vi "Wait for Message.vi"(1 "gui notification":string, 2 "cases to ignore":string[](array[string]), 3 "last state":string, 4 "acquisition state name":string) -> (0 "wait for notification?":bool)   [LabVIEW 2020]
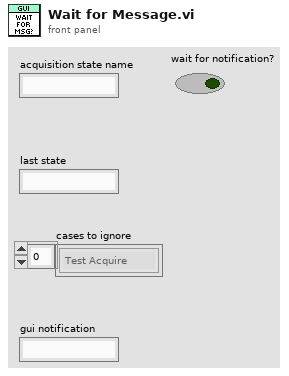
[diagram p1: front panel]
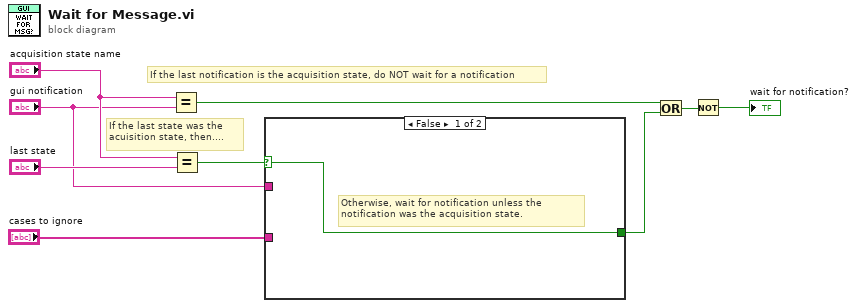
[diagram p0: block diagram]
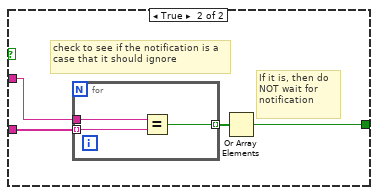
[diagram p2: hidden frame]
diagram:
  # "If the last notification is the acquisition state, do NOT wait for a notification"
  # "If the last state was the acuisition state, then...."
  n1 = Equal?(x="acquisition state name", y="gui notification") -> (x = y?=w9:bool)
  n2 = Equal?(x="acquisition state name", y="last state") -> (x = y?=w2:bool)
  n3 = case shown="False" w2 {
    selector: w2 -> [w10 _]
    tunnel: [w10 w14] -> w8
    tunnel: "cases to ignore" -> [_ w13]
    tunnel: "gui notification" -> [_ w12]
    frame False {
      # "Otherwise, wait for notification unless the notification was the acquisition state."
    }
    frame True {
      # "If it is, then do NOT wait for notification"
      # "check to see if the notification is a case that it should ignore"
      n4 = for {
        tunnel: w13 -> [w17] mode=indexing
        tunnel: w12 -> [w16]
        tunnel: [w15] -> w11 mode=indexing
        n5 = Equal?(x=w16, y=w17) -> (x = y?=w15:bool)
      }
      n6 = Or Array Elements(Boolean array=w11) -> (logical OR=w14:bool)
    }
  }
  n7 = Or(x=w9, y=w8) -> (x .or. y?=w7:bool)
  n8 = Not(x=w7) -> (.not. x?=→"wait for notification?":bool)
